vi "inteference -- find center V22.vi"(7 "number of points":i32, 8 "complex region":T1={"max re"=5.161869466666667e-06, "min re"=5.176843333333334e-06, "max im"=-2.467216e-05, "min im"=-0.001573233, "delta re"=0.003211203, "delta im"=0.00165815, "center re"=0.0015485608400000002, "delta  z"=0.0015530530000000002+0.0i, "center im"=0.0, "center z"=0.0+0.0i, "d im"=0.0, "d re"=0.0, "d z"=0.0+0.0i}, 9 "pond":cdb[][](array[numeric]), 10 "point sources":cdb[](array[numeric]), 11 "wave packet":cdb[][](array[numeric])) -> (2 "z (center)":cdb)   [LabVIEW 2018]
uses:
  complex region.ctl
  <vilib>/Analysis/Matrix/Numeric/Conversions/Array To Matrix - CA2.vi
  <vilib>/Analysis/Matrix/Numeric/Add/Add - CM,CM.vi
  <vilib>/Analysis/Matrix/Numeric/Complex/Complex To Polar - CM.vi
  <vilib>/Analysis/Matrix/NI_Matrix.lvlib
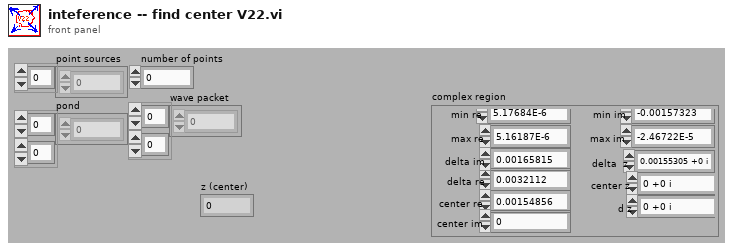
[diagram p1: front panel]
types:
  T1 = typedef "complex region.ctl" = cluster{"max re":dbl, "min re":dbl, "max im":dbl, "min im":dbl, "delta re":dbl, "delta im":dbl, "center re":dbl, "delta  z":cdb, "center im":dbl, "center z":cdb, "d im":dbl, "d re":dbl, "d z":cdb}
  T2 = typedef "NI_Matrix.lvlib/ComplexMatrix.ctl" = cdb[][]
  T3 = typedef "NI_Matrix.lvlib/RealMatrix.ctl" = dbl[][]
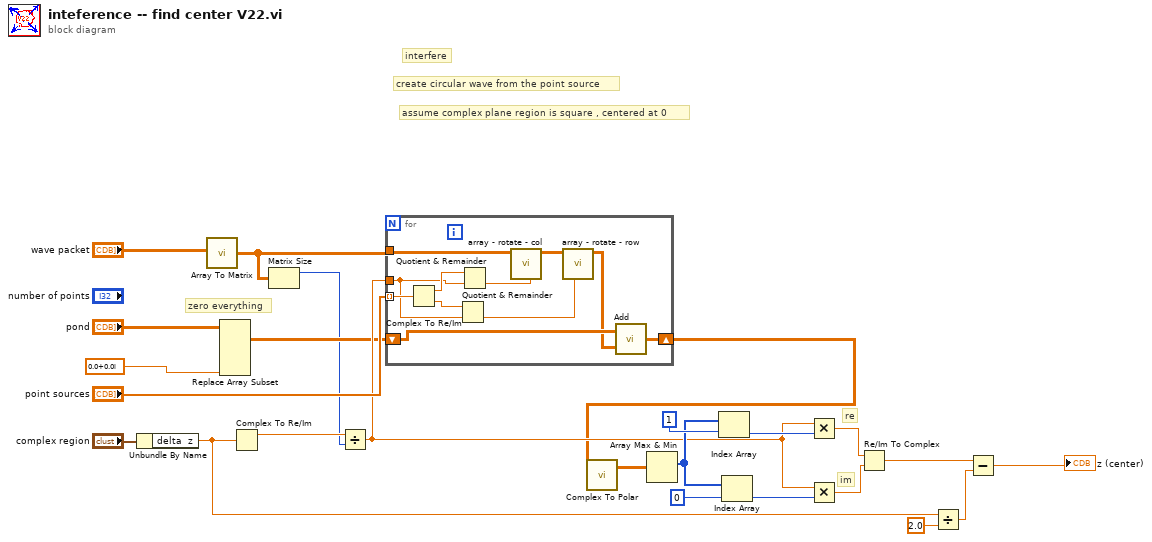
[diagram p0: block diagram]
diagram:
  # "interfere"
  # "create circular wave from the point source"
  # "zero everything"
  # "assume complex plane region is square , centered at 0"
  # "re"
  # "im"
  n1 = Unbundle By Name("complex region") -> ("delta  z"=w12:cdb)
  n2 = call-poly <vilib>:"Array To Matrix.vi"("Complex 2D Array"="wave packet") -> ("Complex Matrix"=w2:T2)
  n3 = Replace Array Subset(array="pond", new element=cdb 0.0+0.0i) -> (w5:T2)  [unwired: 4 in]
  n4 = Complex To Re/Im(x + iy=w12) -> (x=w16:dbl)  [unwired: 1 out]
  n5 = Matrix Size(0:w2) -> (1:w1:i32)  [unwired: 1 out]
  n6 = Divide(x=w16, y=w1) -> (x/y=w8:dbl)
  n7 = for {
    shift-right: [w34] -> w3
    shift-left: w5 -> [w35]
    tunnel: "point sources" -> [w31] mode=indexing
    tunnel: w2 -> [w29]
    tunnel: w8 -> [w30]
    n8 = Complex To Re/Im(x + iy=w31) -> (x=w33:dbl, y=w32:dbl)
    n9 = Quotient & Remainder(x=w32, y=w30) -> (floor(x/y)=w25:dbl)  [unwired: 1 out]
    n10 = Quotient & Remainder(x=w33, y=w30) -> (floor(x/y)=w26:dbl)  [unwired: 1 out]
    n11 = call "array - rotate - col.vi"("rotate column"=w26, "input matrix"=w29) -> ("output matrix"=w28:T2)  [unwired: 9 in]
    n12 = call "array - rotate - row.vi"("rotate row"=w25, "input matrix"=w28) -> ("output matrix"=w27:T2)  [unwired: 9 in]
    n13 = call-poly <vilib>:"Add.vi"("Complex Matrix B"=w27, "Complex Matrix A"=w35) -> ("A + B"=w34:T2)
  }
  n14 = call-poly <vilib>:"Complex To Polar.vi"("Complex Matrix r*e^iQ"=w3) -> ("Modulus r"=w20:T3)  [unwired: 1 out]
  n15 = Array Max & Min(array=w20) -> (max index (indices)=w19:i32[])  [unwired: 3 out]
  n16 = Index Array(array=w19, index=1) -> (element=w18:i32)
  n17 = Index Array(array=w19, index=0) -> (element=w17:i32)
  n18 = Multiply(x=w8, y=w18) -> (x*y=w15:dbl)
  n19 = Multiply(x=w8, y=w17) -> (x*y=w14:dbl)
  n20 = Re/Im To Complex(1:w14, 2:w15) -> (0:w10:cdb)
  n21 = Divide(x=w12, y=2.0) -> (x/y=w11:cdb)
  n22 = Subtract(x=w10, y=w11) -> (x-y=→"z (center)":cdb)
